vi "Search and Replace Pattern.vi"(0 "string":string, 1 "regular expression (\"\")":string, 2 "replace string (\"\")":string, 3 "offset (0)":i32, 4 "replace all? (F)":bool) -> (5 "result string":string, 6 "offset past match":i32)   [LabVIEW 2020]
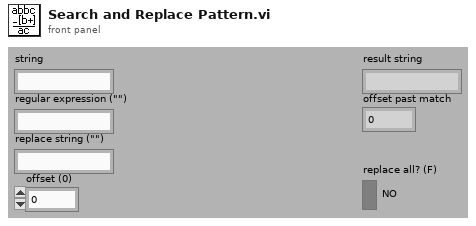
[diagram p1: front panel]
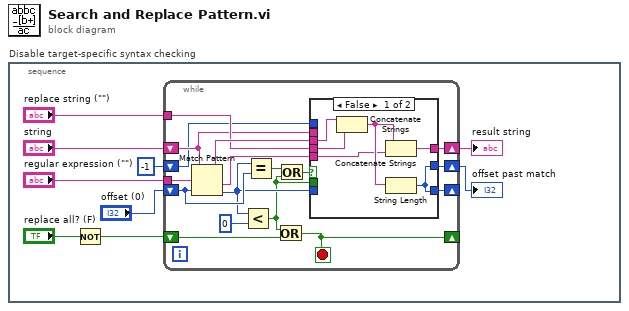
[diagram p0: block diagram]
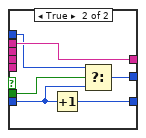
[diagram p2: hidden frame]
diagram:
  n1 = stacked-sequence "Disable target-specific syntax checking" {
    frame #0 {
      n2 = Not(x="replace all? (F)") -> (.not. x?=w5:bool)
      n3 = while {
        shift-right: [w20] -> _
        shift-left: w5 -> [w21]
        shift-right: [w18] -> _
        shift-left: "offset (0)" -> [w14]
        shift-right: [w22] -> w4
        shift-left: "string" -> [w19]
        tunnel: "regular expression (\"\")" -> [w26]
        tunnel: "replace string (\"\")" -> [w23]
        shift-right: [w12] -> w2
        shift-left: -1 -> [w11]
        stop <- w20 stop-if-true
        n4 = Match Pattern(string=w19, regular expression=w26, offset (0)=w14) -> (before substring=w25:string, after substring=w24:string, offset past match=w13:i32)  [unwired: 1 out]
        n5 = Less?(x=w13, y=0) -> (x < y?=w10:bool)
        n6 = Equal?(x=w13, y=w14) -> (x = y?=w15:bool)
        n7 = Or(x=w10, y=w21) -> (x .or. y?=w20:bool)
        n8 = Or(x=w15, y=w10) -> (x .or. y?=w16:bool)
        n9 = case shown="False" w16 {
          tunnel: w25 -> [w31 _]
          tunnel: w24 -> [w28 _]
          tunnel: w23 -> [w30 _]
          tunnel: [w32 w38] -> w22
          tunnel: w19 -> [_ w38]
          tunnel: [w27 w37] -> w18
          tunnel: w13 -> [_ w34]
          tunnel: [w27 w33] -> w12
          tunnel: w11 -> [_ w35]
          tunnel: w10 -> [_ w36]
          frame False {
            n10 = Concatenate Strings(w31, w30) -> (w29:string)
            n11 = Concatenate Strings(w29, w28) -> (w32:string)
            n12 = String Length(string=w29) -> (length=w27:i32)
          }
          frame True {
            n13 = Increment(x=w34) -> (x+1=w37:i32)
            n14 = Select(t=w35, s=w36, f=w34) -> (s? t:f=w33:i32)
          }
        }
      }
      "result string" <- w4
      "offset past match" <- w2
    }
  }
